vi "Show Windows System(MESSAGE-三鍵).vi"(5 "Error Selection":i32(ring) items=["Mode", "-100001", "002", "-100003", "-100004", "-100005", "-100006", "-100007", "-100008", "-100009", "-100010", "-100011", "-100012", "-100013", "-100014", "-100015", "200001", "200002", "200003", "200004", "200005", "200006", "200007", "200008", "200009", "200010", "200011", "200012"], 6 "Error Message Array":string[][](array[string]), 7 "_error In":errorcluster, 9 "Show":bool=TRUE, 10 "vi reference in":refnum<vi>) -> (0 "_error out":errorcluster, 2 "Selection Result":enum16{"Retry", "Reset", "Skip", "Nothing"}(ring), 3 "vi reference out":refnum<vi>)   [LabVIEW 2015]
panel:
  in  "Skip":bool
  in  "Reset":bool
  in  "Retry":bool
  out "Error Message":string
  out "Error Code":string
  in  "Check":bool=TRUE
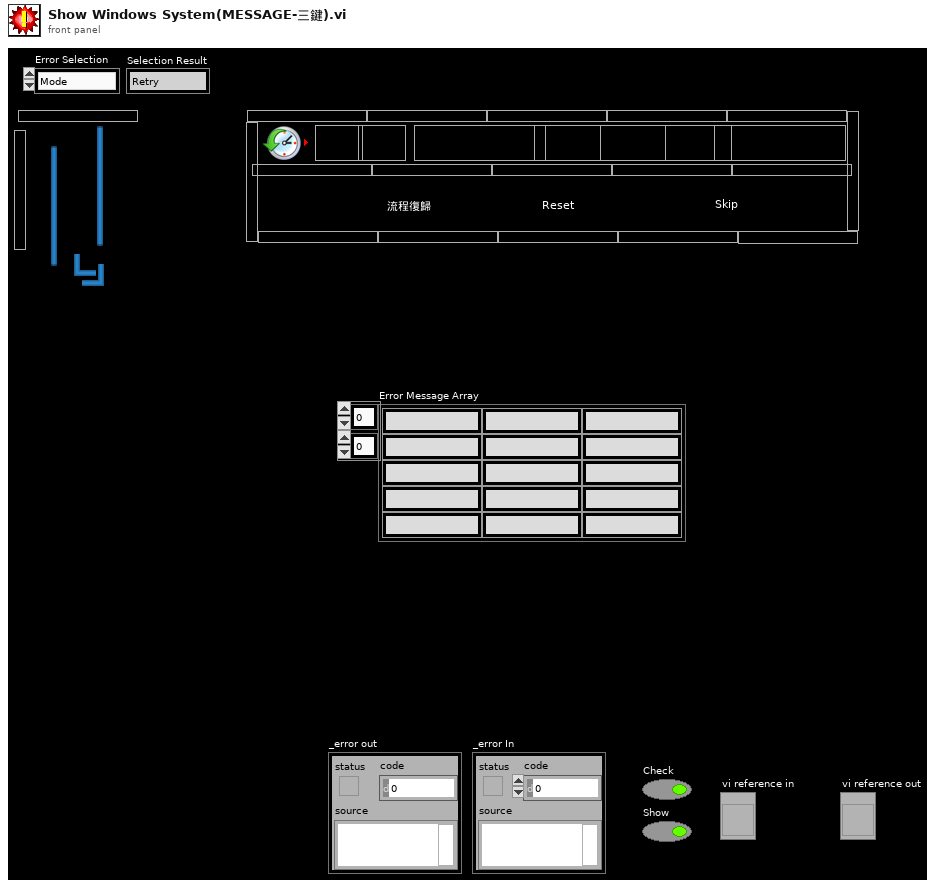
[diagram p1: front panel]
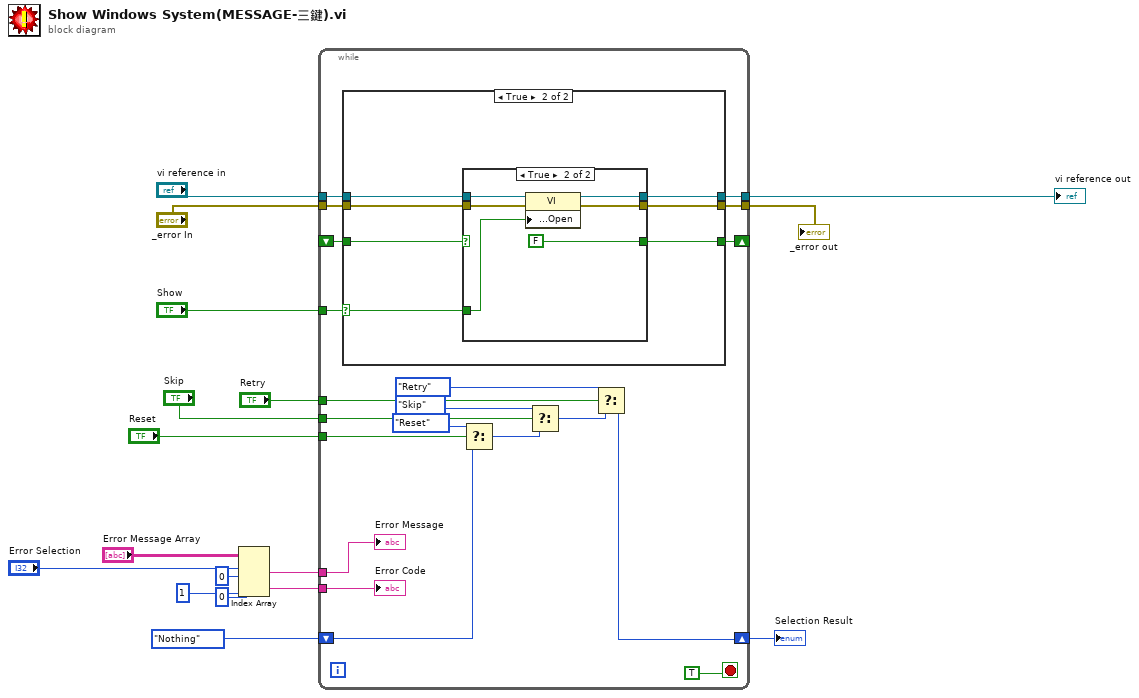
[diagram p0: block diagram]
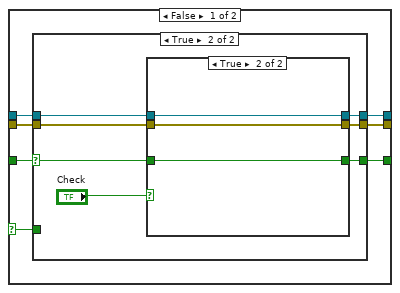
[diagram p2: hidden frame]
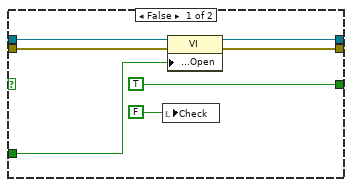
[diagram p3: hidden frame]
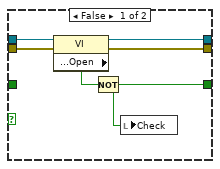
[diagram p4: hidden frame]
diagram:
  n1 = Index Array(array="Error Message Array", index (row) #1="Error Selection", index (col) #1=0 ("disabled index (col)"), index (row) #2=1 ("disabled index (row)"), index (col) #2=0 ("disabled index (col)")) -> (element #1=w13:string, element #2=w8:string)
  n2 = while {
    shift-right: [w33] -> _
    shift-left: _ -> [w32]
    tunnel: "Show" -> [w31]
    tunnel: "vi reference in" -> [w37]
    tunnel: "_error In" -> [w36]
    tunnel: [w35] -> w5
    tunnel: [w34] -> w14
    tunnel: w13 -> [w19]
    shift-right: [w20] -> w11
    shift-left: enum16{"Retry", "Reset", "Skip", "Nothing"}."Nothing" ("Selection Result") -> [w26]
    tunnel: "Retry" -> [w29]
    tunnel: "Skip" -> [w27]
    tunnel: "Reset" -> [w28]
    tunnel: w8 -> [w18]
    stop <- TRUE stop-if-true
    n3 = case shown="True" w31 {
      selector: w31 -> [w38 w68]
      tunnel: w37 -> [w44 w74]
      tunnel: w36 -> [w43 w73]
      tunnel: [w42 w72] -> w35
      tunnel: [w41 w71] -> w34
      tunnel: [w39 w70] -> w33
      tunnel: w32 -> [w40 w69]
      frame False {
        n4 = case shown="True" w40 {
          selector: w40 -> [_ w52]
          tunnel: w44 -> [w51 w58]
          tunnel: w43 -> [w50 w57]
          tunnel: [w49 w56] -> w42
          tunnel: [w48 w55] -> w41
          tunnel: [TRUE w53] -> w39
          tunnel: w38 -> [w46 _]
          frame False {
            n5 = local write "Check"(FALSE ("Check")) -> ()
            n6 = property class="VI"(reference=w51, error in=w50, "Front Panel.Open"=w46) -> (reference out=w49:refnum<vi>, error out=w48:errorcluster)
          }
          frame True {
            n7 = case shown="True" "Check" {
              tunnel: w58 -> [w64 w66]
              tunnel: w57 -> [w63 w65]
              tunnel: [w62 w66] -> w56
              tunnel: [w61 w65] -> w55
              tunnel: [w59 w67] -> w53
              tunnel: w52 -> [_ w67]
              frame False {
                n8 = property class="VI"(reference=w64, error in=w63) -> (reference out=w62:refnum<vi>, error out=w61:errorcluster, "Front Panel.Open"=w60:bool)
                n9 = Not(x=w60) -> (.not. x?=w59:bool)
                n10 = local write "Check"(w59) -> ()
              }
              frame True {
              }
            }
          }
        }
      }
      frame True {
        n11 = case shown="True" w69 {
          selector: w69 -> [w77 _]
          tunnel: w74 -> [w76 w83]
          tunnel: w73 -> [w75 w82]
          tunnel: [w76 w81] -> w72
          tunnel: [w75 w80] -> w71
          tunnel: [w77 FALSE] -> w70
          tunnel: w68 -> [_ w78]
          frame False {
          }
          frame True {
            n12 = property class="VI"(reference=w83, error in=w82, "Front Panel.Open"=w78) -> (reference out=w81:refnum<vi>, error out=w80:errorcluster)
          }
        }
      }
    }
    n13 = Select(t=enum16{"Retry", "Reset", "Skip", "Nothing"}."Reset" ("Selection Result"), s=w28, f=w26) -> (s? t:f=w22:enum16{"Retry", "Reset", "Skip", "Nothing"})
    n14 = Select(t=enum16{"Retry", "Reset", "Skip", "Nothing"}."Skip" ("Selection Result"), s=w27, f=w22) -> (s? t:f=w21:enum16{"Retry", "Reset", "Skip", "Nothing"})
    n15 = Select(t=enum16{"Retry", "Reset", "Skip", "Nothing"}."Retry" ("Selection Result"), s=w29, f=w21) -> (s? t:f=w20:enum16{"Retry", "Reset", "Skip", "Nothing"})
    "Error Code" <- w18
    "Error Message" <- w19
  }
  "_error out" <- w14
  "vi reference out" <- w5
  "Selection Result" <- w11
